vi "mecanum-drive-pose-est-test.vi"(8 "error in (no error)":errorcluster) -> (0 "error out":errorcluster, 3 "Test Passed":bool)   [LabVIEW 2019]
uses:
  <vilib>/Rock Robotics/WPI/ThirdParty/JAS_Junk/TrajLib/MatBuilder_Create.vi
  <vilib>/Rock Robotics/WPI/ThirdParty/JAS_Junk/TrajLib/MatrixHelper_CoerceSize.vi
  <vilib>/Rock Robotics/WPI/ThirdParty/JAS_Junk/TrajLib/Util_CalcDist.vi
  <vilib>/Analysis/1siggen.llb/Gaussian White Noise.vi
  <vilib>/Rock Robotics/WPI/ThirdParty/JAS_Junk/TrajLib/Trajectory_Library.lvlib
panel:
  out "BenchProcessing Timer Per Pass":dbl
  out "BenchTotalTime":dbl
  out "BenchTotalPasses":dbl
  out "MaxErrPassed":bool
  out "TotalPassed":bool
  out "EerrSumNormalized":dbl
  out "Error Sum":dbl
  out "Max Error":dbl
  out "Using Vision":bool
  in  "UseVIsion":bool=TRUE
  out "VIsionUpdates":i32
  out "TotalTImeSecs":dbl
  out "Position Graph":cluster{dbl[], dbl[]}[](graph)
  out "PoesEstCreateErr":errorcluster
  # "< 0.42"
  # "< 0.25"
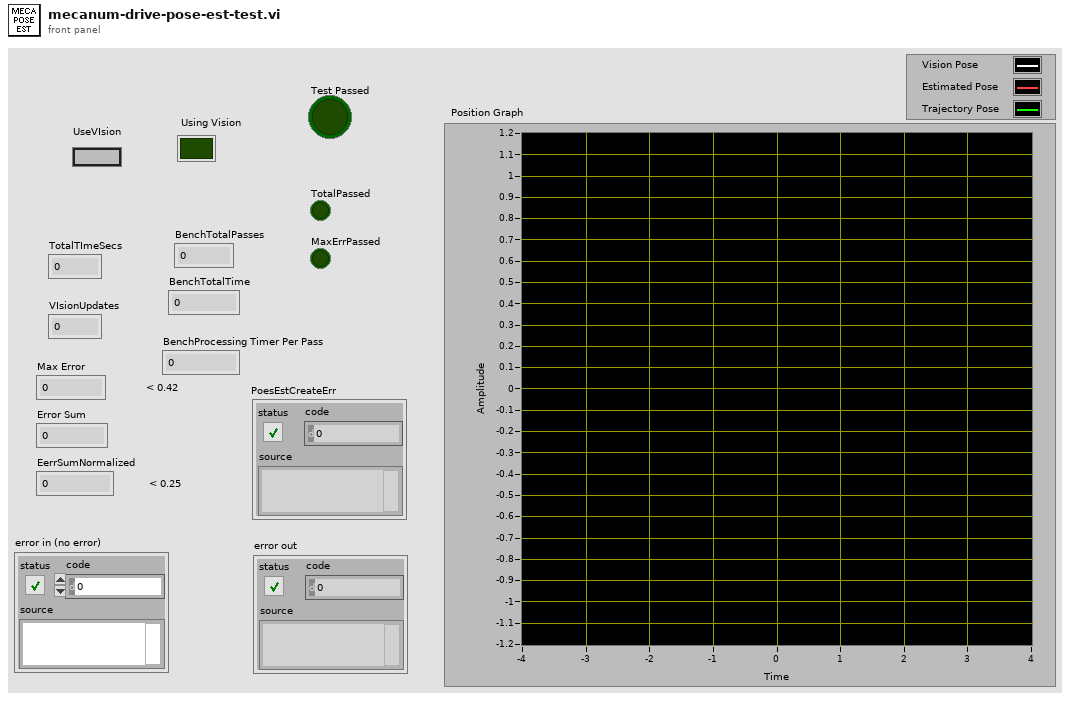
[diagram p1: front panel]
types:
  T1 = typedef "Trajectory_Library.lvlib/TRANSLATION2D.ctl" = cluster{"X":dbl, "Y":dbl}
  T2 = typedef "Trajectory_Library.lvlib/ROTATION2D.ctl" = cluster{"VALUE":dbl, "COS":dbl, "SIN":dbl}
  T3 = typedef "Trajectory_Library.lvlib/POSE2D.ctl" = cluster{"TRANSLATION":T1, "ROTATION":T2}
  T4 = typedef "NI_Matrix.lvlib/RealMatrix.ctl" = dbl[][]
  T5 = typedef "Trajectory_Library.lvlib/MECA_DRIVE_KINEMATICS.ctl" = cluster{"FrontLeft":T1, "FrontRight":T1, "RearLeft":T1, "RearRight":T1, "InverseKinematics":T4, "ForwardKinematics":T4, "PrevCoR":T1}
  T6 = typedef "Trajectory_Library.lvlib/TRAJ_CONFIG.ctl" = cluster{"MaxVelocity":dbl, "Max Acceleration":dbl, "StartVelocity":dbl, "End Velocity":dbl, "Reversed":bool, "DiffDrKineConstntDefined":bool, "CentAcellConstntDefined":bool, "DiffDrVoltConstntDefined":bool, "DIFF_DRIVE_KINE_CONSTRAINT":T7, "CENTRIPETAL_ACCEL_CONSTRAINT":T9, "SwerveDrKineConstntDefined":bool, "SWERVE_DRIVE_KINE_CONSTRAINT":T10, "DIFF_DRIVE_VOLTAGE_CONSTRAINT":T12, "MECANUM_DRIVE_KINE_CONSTRAINT":T14, "MecanumDrKineConstntDefined":bool}
  T7 = typedef "Trajectory_Library.lvlib/TRAJ_CONSTRAINT_DIIF_DRIVE_KINEMATICS.ctl" = cluster{"Max Speed (M/S)":dbl, "DIFF_DRIVE_KINEMATICS":T8, "Max Accel (M/S2)":dbl}
  T8 = typedef "Trajectory_Library.lvlib/DIFF_DRIVE_KINEMATICS.ctl" = cluster{"TrackWidth_Meters":dbl}
  T9 = typedef "Trajectory_Library.lvlib/TRAJ_CONSTRAINT_CENTRIPETAL_ACCEL.ctl" = cluster{"Max Cent Accel":dbl}
  T10 = typedef "Trajectory_Library.lvlib/TRAJ_CONSTRAINT_SWERVE_DRIVE_KINEMATICS.ctl" = cluster{"Max Speed (M/S)":dbl, "SwerveKinematics":T11}
  T11 = typedef "Trajectory_Library.lvlib/SWERVE_DRIVE_KINEMATICS.ctl" = cluster{"NumModules":i32, "InverseKinematics":T4, "ForwardKinematics":T4, "Modules":T1[], "PrevCoR":T1}
  T12 = typedef "Trajectory_Library.lvlib/TRAJ_CONSTRAINT_DIIF_DRIVE_VOLTAGE.ctl" = cluster{"Max Voltage":dbl, "DIFF_DRIVE_KINEMATICS":T8, "SIMPLE_MOTOR_FF":T13}
  T13 = typedef "Trajectory_Library.lvlib/SIMPLE_MOTOR_FF.ctl" = cluster{"Ks":dbl, "Kv":dbl, "Ka":dbl}
  T14 = typedef "Trajectory_Library.lvlib/TRAJ_CONSTRAINT_MECA_DRIVE_KINEMATICS.ctl" = cluster{"Max Speed (M/S)":dbl, "MECA_DRIVE_KINEMATICS":T5}
  T15 = typedef "Trajectory_Library.lvlib/MECA_DRIVE_POSE_EST.ctl" = cluster{"M_VisionContR":T4, "m_nominal_dT":dbl, "m_PrevTime_Sec":dbl, "m_GyroOffset":T2, "m_PrevAngle":T2, "m_Observer":T16, "m_kinematics":T5, "Pose_Buffer":T19}
  T16 = typedef "Trajectory_Library.lvlib/UNSCENTED_KALMAN_FILTER.ctl" = cluster{"m_P":T4, "m_xHat":T4, "States":i32, "Outputs":i32, "m_ContR":T4, "m_ContQ":T4, "m_SigmasF":T4, "m_dT_Sec":dbl, "MERWE_SCALED_SIGMA_PTS":T17, "meanFuncX":T18, "meanFuncY":T18, "residualFuncX":T18, "residualFuncY":T18, "addFuncX":T18, "addFuncXExtra":variant, "residualFuncYExtra":variant, "residualFuncXExtra":variant, "MeanFuncYExtra":variant, "MeanFuncXExtra":variant, "Inputs":i32}
  T17 = typedef "Trajectory_Library.lvlib/MERWE_SCALED_SIGMA_PTS.ctl" = cluster{"m_Wm":T4, "States":i32, "Alpha":dbl, "m_Wc":T4, "Kappa":i32}
  T18 = typedef "Trajectory_Library.lvlib/CALLBACK_FUNC_TYPE.ctl" = refnum<vi>
  T19 = typedef "Trajectory_Library.lvlib/TIME_INTERPOLATABLE_POSE.ctl" = cluster{"TimeStamps":dbl[], "Pose":T3[], "Min_TimeStamp":dbl, "Max_TimeStamp":dbl, "ItemCount":i32, "MaxBufferTime":dbl}
  T20 = typedef "Trajectory_Library.lvlib/TRAJECTORY.ctl" = cluster{"TotalTImeSecs":dbl, "States":T21[]}
  T21 = typedef "Trajectory_Library.lvlib/TRAJ_STATE.ctl" = cluster{"TimeSeconds":dbl, "Velocity":dbl, "Acceleration":dbl, "POSE":T3, "Curvature":dbl}
  T22 = typedef "Trajectory_Library.lvlib/CHASSIS_SPEEDS.ctl" = cluster{"vX":dbl, "vY":dbl, "vOmega":dbl}
  T23 = typedef "Trajectory_Library.lvlib/MECA_WHEEL_SPEEDS.ctl" = cluster{"FrontLeftSpeed":dbl, "FrontRightSpeed":dbl, "RearLeftSpeed":dbl, "RearRightSpeed":dbl}
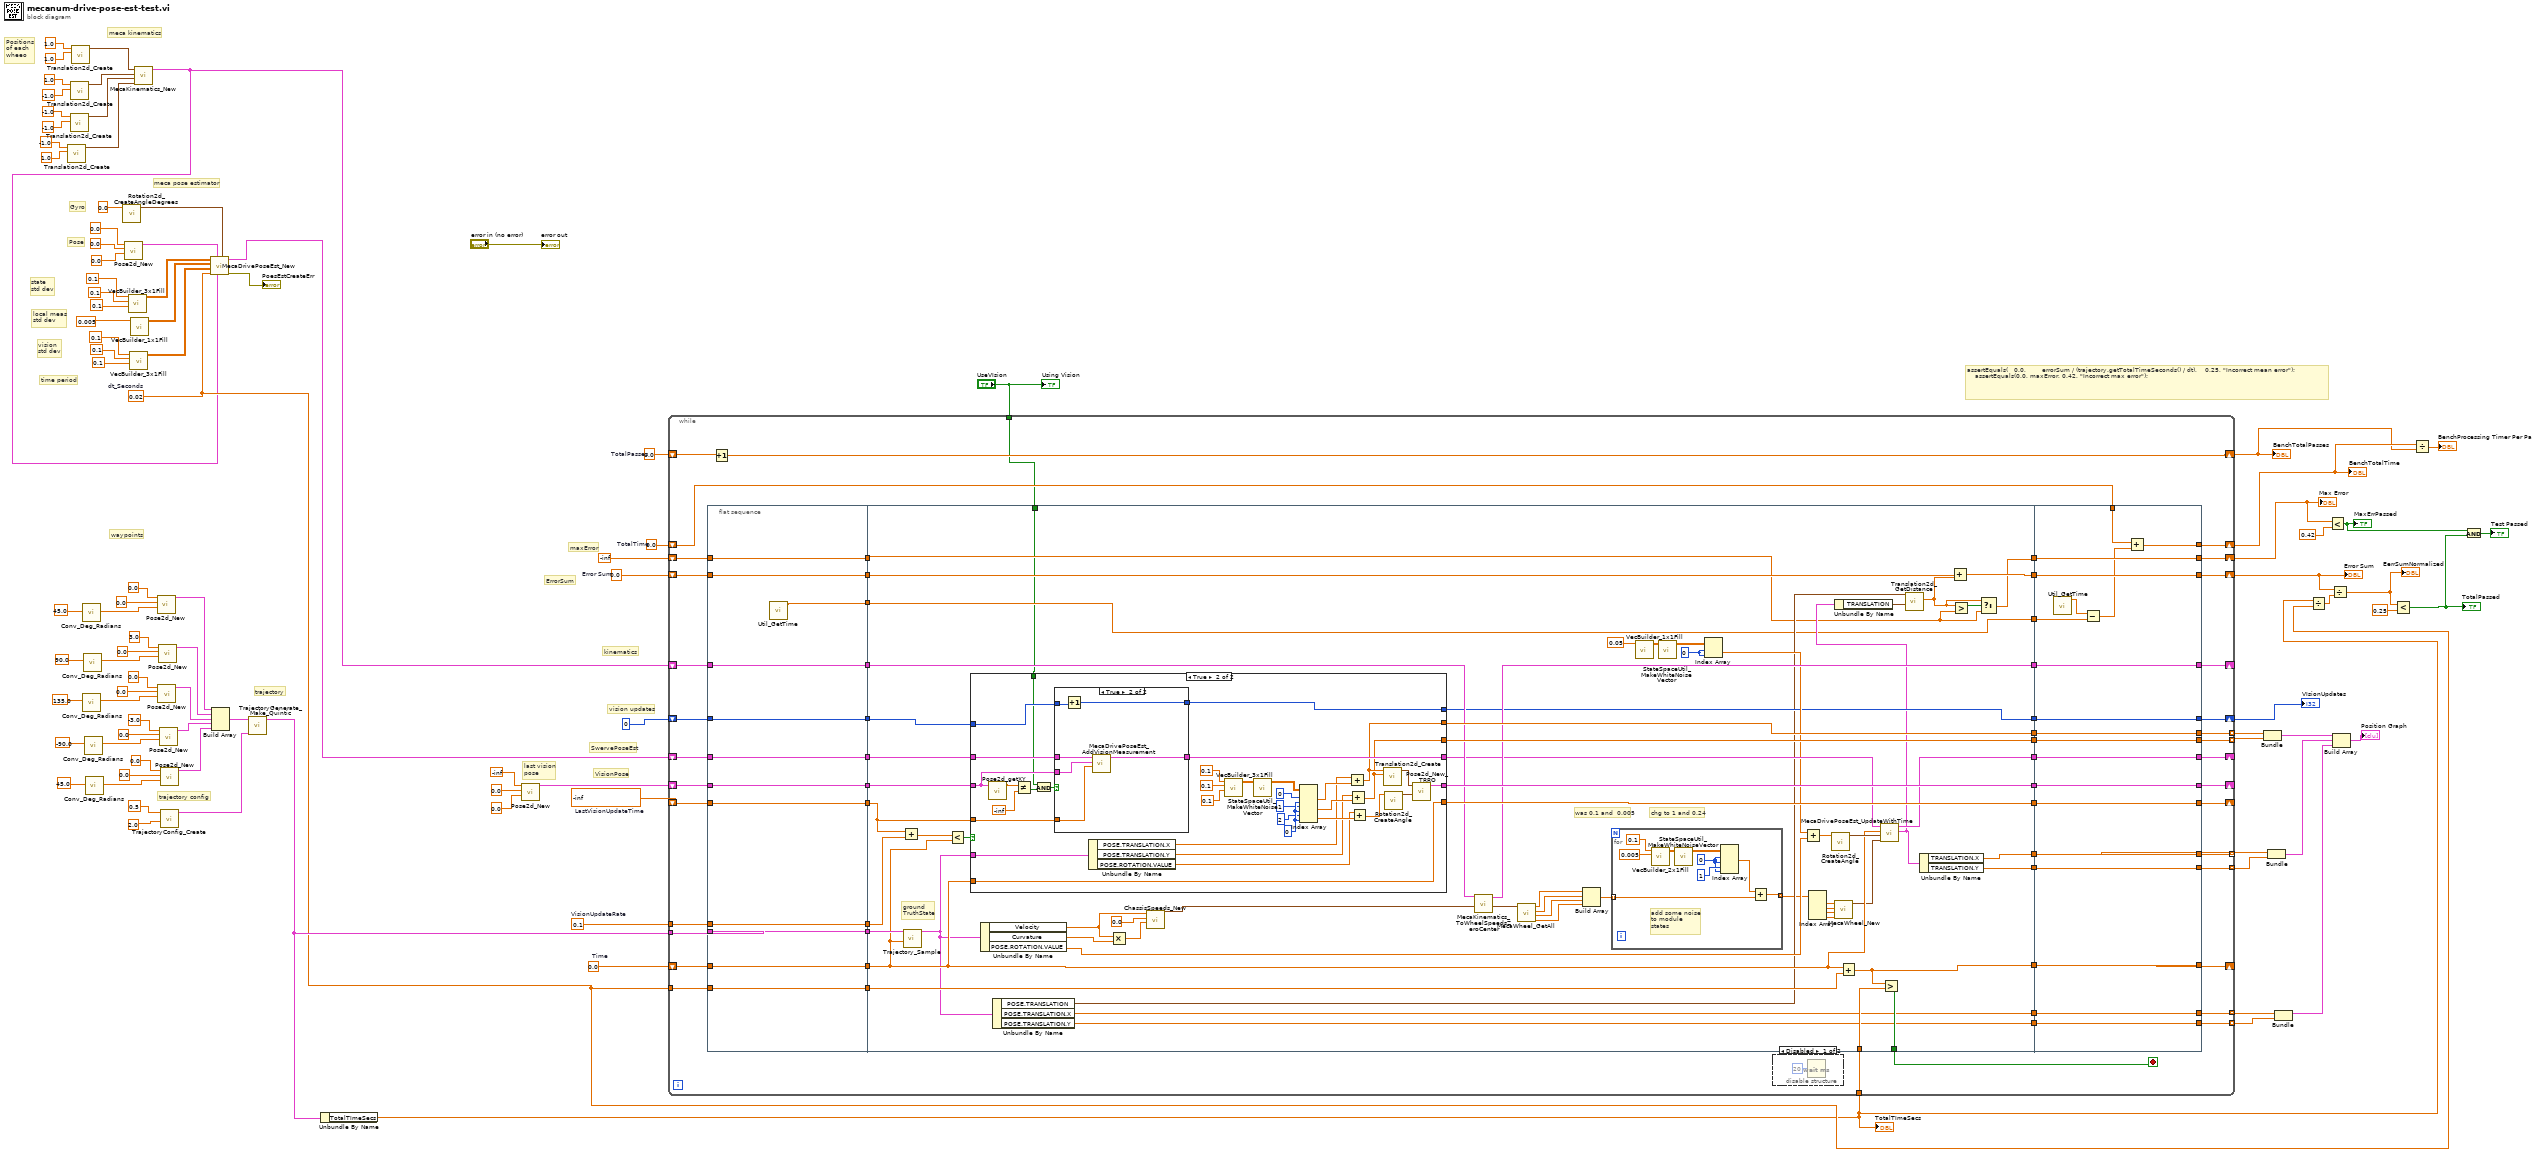
[diagram p0: block diagram]
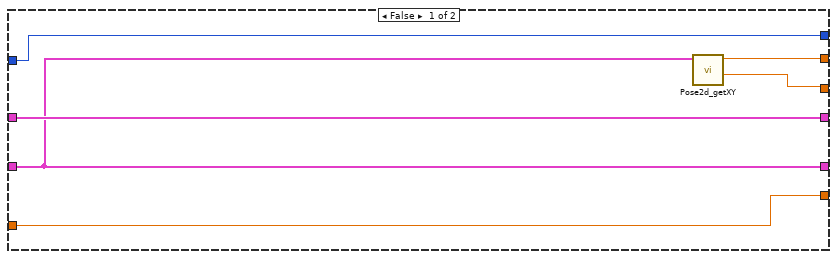
[diagram p3: hidden frame]
diagram:
  w8 = 0.0  # TotalPasses
  w9 = 0.0  # TotalTime
  w21 = 0.0  # Error Sum
  w39 = 0.1  # VisionUpdateRate
  w40 = -inf  # LastVisionUpdateTime
  w42 = 0.0  # Time
  w19 = 0.02  # dt_Seconds
  # "assertEquals(   0.0,        errorSum / (trajectory.getTotalTimeSeconds() / dt),    0.25, \"Incorrect mean error\");\n    assertEquals(0.0, maxError, 0.42, \"Incorrect max error\");"
  # "ErrorSum"
  # "maxError"
  # "vision updates"
  # "kinematics"
  # "SwervePoseEst"
  # "VisionPose"
  # "last vision\npose"
  # "time period"
  # "vision \nstd dev"
  # "local meas\nstd dev"
  # "state\nstd dev"
  # "Pose"
  # "Gyro"
  # "Positions\nof each\nwheeo"
  # "meca pose estimator"
  # "meca kinematics"
  # "trajectory config"
  # "trajectory"
  # "waypoints"
  n1 = call <vilib>:"Translation2d_Create.vi"("Y"=1.0, "X"=-1.0) -> ("TRANSLATION"=w60:T1)  [unwired: 9 in]
  n2 = call <vilib>:"Translation2d_Create.vi"("Y"=-1.0, "X"=-1.0) -> ("TRANSLATION"=w61:T1)  [unwired: 9 in]
  n3 = call <vilib>:"Translation2d_Create.vi"("Y"=-1.0, "X"=1.0) -> ("TRANSLATION"=w62:T1)  [unwired: 9 in]
  n4 = call <vilib>:"Translation2d_Create.vi"("Y"=1.0, "X"=1.0) -> ("TRANSLATION"=w63:T1)  [unwired: 9 in]
  n5 = call <vilib>:"Conv_Deg_Radians.vi"("Degress"=45.0 ("Heading")) -> ("Radians"=w77:dbl)  [unwired: 10 in]
  n6 = call <vilib>:"Conv_Deg_Radians.vi"("Degress"=135.0 ("Heading")) -> ("Radians"=w85:dbl)  [unwired: 10 in]
  n7 = call <vilib>:"Conv_Deg_Radians.vi"("Degress"=90.0 ("Heading")) -> ("Radians"=w81:dbl)  [unwired: 10 in]
  n8 = call <vilib>:"Conv_Deg_Radians.vi"("Degress"=-90.0 ("Heading")) -> ("Radians"=w89:dbl)  [unwired: 10 in]
  n9 = call <vilib>:"Conv_Deg_Radians.vi"("Degress"=45.0 ("Heading")) -> ("Radians"=w93:dbl)  [unwired: 10 in]
  n10 = call <vilib>:"Rotation2d_CreateAngleDegrees.vi"("Angle_Degrees"=0.0) -> ("ROTATION"=w59:T2)  [unwired: 10 in]
  n11 = call <vilib>:"Pose2d_New.vi"("Heading"=0.0, "Y"=0.0, "X"=0.0) -> ("out POSe"=w57:T3)  [unwired: 8 in]
  n12 = call <vilib>:"VecBuilder_3x1Fill.vi"("R2"=0.1 ("element"), "R1"=0.1 ("element"), "R0"=0.1 ("element")) -> ("output matrix"=w49:T4)  [unwired: 8 in]
  n13 = call <vilib>:"VecBuilder_3x1Fill.vi"("R2"=0.1 ("element"), "R1"=0.1 ("element"), "R0"=0.1 ("element")) -> ("output matrix"=w44:T4)  [unwired: 8 in]
  n14 = call <vilib>:"VecBuilder_1x1Fill.vi"("R0_C0"=0.005 ("element")) -> ("output matrix"=w48:T4)  [unwired: 10 in]
  n15 = call <vilib>:"MecaKinematics_New.vi"("RearRight"=w60, "RearLeft"=w61, "FrontRight"=w62, "FrontLeft"=w63) -> ("MECA_DRIVE_KINEMATICS"=w1:T5)  [unwired: 7 in]
  n16 = call <vilib>:"Pose2d_New.vi"("Heading"=w77, "Y"=0.0, "X"=0.0) -> ("out POSe"=w76:T3)  [unwired: 8 in]
  n17 = call <vilib>:"Pose2d_New.vi"("Heading"=w85, "Y"=0.0, "X"=0.0) -> ("out POSe"=w73:T3)  [unwired: 8 in]
  n18 = call <vilib>:"Pose2d_New.vi"("Heading"=w81, "Y"=0.0, "X"=3.0) -> ("out POSe"=w74:T3)  [unwired: 8 in]
  n19 = call <vilib>:"Pose2d_New.vi"("Heading"=w89, "Y"=0.0, "X"=-3.0) -> ("out POSe"=w72:T3)  [unwired: 8 in]
  n20 = call <vilib>:"Pose2d_New.vi"("Heading"=w93, "Y"=0.0, "X"=0.0) -> ("out POSe"=w98:T3)  [unwired: 8 in]
  n21 = call <vilib>:"TrajectoryConfig_Create.vi"("MaxAcceleration"=2.0, "MaxVelocity"=0.5) -> ("TRAJECTORY_CONFIG"=w95:T6)  [unwired: 9 in]
  n22 = call <vilib>:"MecaDrivePoseEst_New.vi"("gyroAngle"=w59, "MecanumKinematics"=w1, "InitialPose"=w57, "dt_Seconds"=w19, "VisionMeasurementStdDevs"=w44, "LocalMeasurementStdDevs"=w48, "StateStdDevs"=w49) -> ("Error"=→"PoesEstCreateErr":errorcluster, "MecaDrivePoseEstimate"=w2:T15)  [unwired: 3 in]
  n23 = Build Array(w76, w74, w73, w72, w98) -> (w96:T3[])
  n24 = call <vilib>:"TrajectoryGenerate_Make_Quintic.vi"("traj_config"=w95, "waypointPOSE"=w96) -> ("TRAJECTORY"=w41:T20)  [unwired: 8 in, 1 out]
  n25 = Unbundle By Name(w41) -> ("TotalTImeSecs"=w12:dbl)
  "TotalTImeSecs" <- w12
  n26 = call <vilib>:"Pose2d_New.vi"("Heading"=0.0, "Y"=0.0, "X"=-inf) -> ("out POSe"=w35:T3)  [unwired: 8 in]
  n27 = while {
    tunnel: w19 -> [w159]
    shift-right: [w158] -> _
    shift-left: w42 -> [w145]
    tunnel: w41 -> [w156]
    tunnel: w12 -> [w157]
    shift-right: [w150] -> _
    shift-left: w40 -> [w152]
    tunnel: w39 -> [w155]
    shift-right: [w151] -> _
    shift-left: w35 -> [w154]
    shift-right: [w144] -> _
    shift-left: w2 -> [w153]
    tunnel: [w149] -> w34 mode=indexing
    tunnel: [w148] -> w33 mode=indexing
    shift-right: [w146] -> _
    shift-left: w1 -> [w147]
    tunnel: [w143] -> w32 mode=indexing
    tunnel: [w142] -> w31 mode=indexing
    shift-right: [w140] -> w26
    shift-left: 0 -> [w141]
    tunnel: [w139] -> w25 mode=indexing
    tunnel: [w138] -> w24 mode=indexing
    shift-right: [w135] -> w17
    shift-left: -inf -> [w134]
    shift-right: [w136] -> w20
    shift-left: w21 -> [w137]
    shift-right: [w105] -> w7
    shift-left: w9 -> [w104]
    shift-right: [w102] -> w6
    shift-left: w8 -> [w103]
    tunnel: "UseVIsion" -> [w101]
    stop <- w133 stop-if-true
    n28 = flat-sequence {
      tunnel: w134 -> [w162]
      tunnel: w137 -> [w163]
      tunnel: w141 -> [w164]
      tunnel: w145 -> [w165]
      tunnel: w147 -> [w166]
      tunnel: w152 -> [w167]
      tunnel: w153 -> [w168]
      tunnel: w154 -> [w169]
      tunnel: w155 -> [w170]
      tunnel: w156 -> [w171]
      tunnel: w159 -> [w172]
      tunnel: [w172] -> w132
      tunnel: [w171] -> w131
      tunnel: [w170] -> w130
      tunnel: [w169] -> w129
      tunnel: [w168] -> w128
      tunnel: [w167] -> w127
      tunnel: [w166] -> w126
      tunnel: [w165] -> w125
      tunnel: [w164] -> w124
      tunnel: [w163] -> w123
      tunnel: [w162] -> w122
      tunnel: [w161] -> w107
      tunnel: [w234] -> w133
      tunnel: w157 -> [w232]
      tunnel: w132 -> [w235]
      tunnel: w131 -> [w231]
      tunnel: w130 -> [w229]
      tunnel: w129 -> [w227]
      tunnel: w128 -> [w226]
      tunnel: w127 -> [w225]
      tunnel: w126 -> [w215]
      tunnel: w125 -> [w204]
      tunnel: w124 -> [w200]
      tunnel: w123 -> [w192]
      tunnel: w122 -> [w187]
      tunnel: [w233] -> w121
      tunnel: [w224] -> w120
      tunnel: [w223] -> w119
      tunnel: [w222] -> w118
      tunnel: [w221] -> w117
      tunnel: [w214] -> w116
      tunnel: [w203] -> w115
      tunnel: [w202] -> w114
      tunnel: [w201] -> w113
      tunnel: [w199] -> w112
      tunnel: [w197] -> w111
      tunnel: [w196] -> w110
      tunnel: [w191] -> w109
      tunnel: [w188] -> w108
      tunnel: w107 -> [w186]
      tunnel: [w186] -> w106
      tunnel: w101 -> [w185]
      tunnel: [w298] -> w135
      tunnel: [w299] -> w136
      tunnel: [w300] -> w138
      tunnel: [w301] -> w139
      tunnel: [w302] -> w140
      tunnel: [w303] -> w142
      tunnel: [w304] -> w143
      tunnel: [w305] -> w144
      tunnel: [w306] -> w146
      tunnel: [w307] -> w148
      tunnel: [w308] -> w149
      tunnel: [w309] -> w150
      tunnel: [w310] -> w151
      tunnel: [w311] -> w158
      tunnel: w121 -> [w311]
      tunnel: w120 -> [w310]
      tunnel: w119 -> [w309]
      tunnel: w118 -> [w308]
      tunnel: w117 -> [w307]
      tunnel: w116 -> [w306]
      tunnel: w115 -> [w305]
      tunnel: w114 -> [w304]
      tunnel: w113 -> [w303]
      tunnel: w112 -> [w302]
      tunnel: w111 -> [w301]
      tunnel: w110 -> [w300]
      tunnel: w109 -> [w299]
      tunnel: w108 -> [w298]
      tunnel: w106 -> [w296]
      tunnel: [w295] -> w105
      tunnel: w104 -> [w293]
      frame #0 {
        n29 = call <vilib>:"Util_GetTime.vi"() -> ("FPGA_Time_Seconds"=w161:dbl)  [unwired: 10 in, 1 out]
      }
      frame #1 {
        w209 = 0 ("index (col)")
        # "chg to 1 and 0.24"
        # "was 0.1 and  0.005"
        # "ground\nTruthState"
        n30 = Add(x=w225, y=w229) -> (x+y=w228:dbl)
        n31 = call <vilib>:"Trajectory_Sample.vi"("Time"=w204, "InputTRAJECTORY"=w231) -> ("OutputTRAJ_STATE"=w198:T21)  [unwired: 9 in]
        n32 = Less?(x=w228, y=w204) -> (x < y?=w230:bool)
        n33 = case shown="True" w230 {
          tunnel: w227 -> [w248 w281]
          tunnel: w226 -> [w250 w282]
          tunnel: [w250 w280] -> w213
          tunnel: w225 -> [w249 w279]
          tunnel: w198 -> [_ w272]
          tunnel: [w248 w278] -> w224
          tunnel: w204 -> [_ w258]
          tunnel: [w249 w258] -> w223
          tunnel: [w247 w257] -> w222
          tunnel: [w246 w256] -> w221
          tunnel: w200 -> [w245 w255]
          tunnel: [w245 w254] -> w199
          tunnel: w185 -> [_ w251]
          frame False {
            n34 = call <vilib>:"Pose2d_getXY.vi"("in POSE"=w248) -> ("Y"=w246:dbl, "X"=w247:dbl)  [unwired: 9 in]
          }
          frame True {
            w269 = 0 ("index (col)")
            n35 = call <vilib>:"Pose2d_getXY.vi"("in POSE"=w281) -> ("X"=w284:dbl)  [unwired: 9 in, 1 out]
            n36 = Not Equal?(x=w284, y=-inf) -> (x != y?=w252:bool)
            n37 = And(x=w251, y=w252) -> (x .and. y?=w253:bool)
            n38 = case shown="True" w253 {
              tunnel: w282 -> [w286 w292]
              tunnel: w281 -> [_ w291]
              tunnel: [w286 w290] -> w280
              tunnel: w279 -> [_ w289]
              tunnel: w255 -> [w285 w288]
              tunnel: [w285 w287] -> w254
              frame False {
              }
              frame True {
                n39 = Increment(x=w288) -> (x+1=w287:i32)
                n40 = call <vilib>:"MecaDrivePoseEst_AddVisionMeasurement.vi"("TImeStamp_Seconds"=w289, "visionRobotPose"=w291, "in MecaDrivePoseEstimate"=w292) -> ("OutMecaDrivePoseEstimate"=w290:T15)  [unwired: 7 in, 1 out]
              }
            }
            n41 = Unbundle By Name(w272) -> ("POSE.TRANSLATION.X"=w261:dbl, "POSE.TRANSLATION.Y"=w260:dbl, "POSE.ROTATION.VALUE"=w259:dbl)
            n42 = call <vilib>:"VecBuilder_3x1Fill.vi"("R2"=0.1, "R1"=0.1, "R0"=0.1) -> ("output matrix"=w276:T4)  [unwired: 8 in]
            n43 = call <vilib>:"StateSpaceUtil_MakeWhiteNoiseVector.vi"("StdDevs"=w276) -> ("WhiteNoise"=w270:T4)  [unwired: 9 in, 1 out]
            n44 = Index Array(array=w270, index (row) #1=0 ("index (col)"), index (col) #1=w269, index (row) #2=1 ("index (col)"), index (col) #2=w269, index (row) #3=2 ("index (col)"), index (col) #3=w269) -> (element #1=w263:dbl, element #2=w264:dbl, element #3=w265:dbl)
            n45 = Add(x=w261, y=w263) -> (x+y=w257:dbl)
            n46 = Add(x=w260, y=w264) -> (x+y=w256:dbl)
            n47 = Add(x=w259, y=w265) -> (x+y=w262:dbl)
            n48 = call <vilib>:"Translation2d_Create.vi"("Y"=w256, "X"=w257) -> ("TRANSLATION"=w277:T1)  [unwired: 9 in]
            n49 = call <vilib>:"Rotation2d_CreateAngle.vi"("Angle"=w262) -> ("ROTATION"=w271:T2)  [unwired: 10 in]
            n50 = call <vilib>:"Pose2d_New_TRRO.vi"("ROTATION"=w271, "TRANSLATION"=w277) -> ("outPOSE"=w278:T3)  [unwired: 9 in]
          }
        }
        n51 = Unbundle By Name(w198) -> ("Velocity"=w218:dbl, "Curvature"=w219:dbl, "POSE.ROTATION.VALUE"=w208:dbl)
        n52 = Unbundle By Name(w198) -> ("POSE.TRANSLATION"=w195:T1, "POSE.TRANSLATION.X"=w196:dbl, "POSE.TRANSLATION.Y"=w197:dbl)
        n53 = Multiply(x=w218, y=w219) -> (x*y=w217:dbl)
        n54 = call <vilib>:"ChassisSpeeds_New.vi"("vAngular"=w217, "vY"=0.0, "vX"=w218) -> ("CHASSIS"=w216:T22)  [unwired: 8 in]
        n55 = call <vilib>:"MecaKinematics_ToWheelSpeedsZeroCenter.vi"("ChassisSpeeds"=w216, "in MECA_DRIVE_KINEMATICS"=w215) -> ("MECA_WHEEL_SPEEDS"=w184:T23, "out MECA_DRIVE_KINEMATICS"=w214:T5)  [unwired: 8 in]
        n56 = call <vilib>:"MecaWheel_GetAll.vi"("MECA_WHEEL_SPEEDS"=w184) -> ("RearRightSpeed"=w180:dbl, "RearLeftSpeed"=w181:dbl, "FrontRightSpeed"=w182:dbl, "FrontLeftSpeed"=w183:dbl)  [unwired: 7 in]
        n57 = Build Array(w183, w182, w181, w180) -> (w179:dbl[])
        n58 = for {
          tunnel: [w236] -> w178 mode=indexing
          tunnel: w179 -> [w237] mode=indexing
          w239 = 0 ("index (col)")
          # "add some noise\nto module\nstates"
          n59 = call <vilib>:"VecBuilder_2x1Fill.vi"("R1"=0.005, "R0"=0.1) -> ("output matrix"=w244:T4)  [unwired: 9 in]
          n60 = call <vilib>:"StateSpaceUtil_MakeWhiteNoiseVector.vi"("StdDevs"=w244) -> ("WhiteNoise"=w241:T4)  [unwired: 9 in, 1 out]
          n61 = Index Array(array=w241, index (row) #1=w239, index (col) #1=w239, index (row) #2=1 ("index (col)"), index (col) #2=w239) -> (element #1=w238:dbl)  [unwired: 1 out]
          n62 = Add(x=w238, y=w237) -> (x+y=w236:dbl)
        }
        n63 = call <vilib>:"VecBuilder_1x1Fill.vi"("R0_C0"=0.05 ("R0")) -> ("output matrix"=w212:T4)  [unwired: 10 in]
        n64 = call <vilib>:"StateSpaceUtil_MakeWhiteNoiseVector.vi"("StdDevs"=w212) -> ("WhiteNoise"=w210:T4)  [unwired: 9 in, 1 out]
        n65 = Index Array(array=w210, index (row)=w209, index (col)=w209) -> (element=w207:dbl)
        n66 = Add(x=w207, y=w208) -> (x+y=w206:dbl)
        n67 = Index Array(array=w178) -> (element #1=w176:dbl, element #2=w175:dbl, element #3=w174:dbl, element #4=w173:dbl)  [unwired: 4 in]
        n68 = call <vilib>:"Rotation2d_CreateAngle.vi"("Angle"=w206) -> ("ROTATION"=w205:T2)  [unwired: 10 in]
        n69 = call <vilib>:"MecaWheel_New.vi"("RearRightSpeed"=w173, "RearLeftSpeed"=w174, "FrontRightSpeed"=w175, "FrontLeftSpeed"=w176) -> ("MECA_WHEEL_SPEEDS"=w177:T23)  [unwired: 7 in]
        n70 = Add(x=w204, y=w235) -> (x+y=w233:dbl)
        n71 = call <vilib>:"MecaDrivePoseEst_UpdateWithTime.vi"("MecanumWheelSpeeds"=w177, "GyroAngle"=w205, "CurrentTimeSeconds"=w204, "in MecaDrivePoseEstimate"=w213) -> ("Estimated Pose"=w194:T3, "Out MecaDrivePoseEstimate"=w203:T15)  [unwired: 5 in, 1 out]
        n72 = Unbundle By Name(w194) -> ("TRANSLATION"=w193:T1)
        n73 = Greater?(x=w233, y=w232) -> (0:w234:bool)
        n74 = call <vilib>:"Translation2d_GetDistance.vi"("other Translation"=w193, "In Translation"=w195) -> ("Distance"=w189:dbl)  [unwired: 9 in]
        n75 = Unbundle By Name(w194) -> ("TRANSLATION.X"=w202:dbl, "TRANSLATION.Y"=w201:dbl)
        n76 = Add(x=w192, y=w189) -> (x+y=w191:dbl)
        n77 = Greater?(x=w189, y=w187) -> (0:w190:bool)
        n78 = Select(t=w189, s=w190, f=w187) -> (s? t:f=w188:dbl)
      }
      frame #2 {
        n79 = call <vilib>:"Util_GetTime.vi"() -> ("FPGA_Time_Seconds"=w297:dbl)  [unwired: 10 in, 1 out]
        n80 = Subtract(x=w297, y=w296) -> (x-y=w294:dbl)
        n81 = Add(x=w293, y=w294) -> (x+y=w295:dbl)
      }
    }
    n82 = Increment(x=w103) -> (x+1=w102:dbl)
    n83 = disable-structure shown="Disabled" {
      frame Disabled {
        n84 = Wait (ms)(milliseconds to wait=u32 20) -> ()  [unwired: 1 out]
      }
      frame Enabled {
      }
    }
  }
  "VIsionUpdates" <- w26
  "Max Error" <- w17
  "Error Sum" <- w20
  "BenchTotalPasses" <- w6
  "BenchTotalTime" <- w7
  n85 = Bundle(w34, w33) -> (w30:cluster{dbl[], dbl[]})  [unwired: 1 in]
  n86 = Bundle(w32, w31) -> (w29:cluster{dbl[], dbl[]})  [unwired: 1 in]
  n87 = Bundle(w24, w25) -> (w23:cluster{dbl[], dbl[]})  [unwired: 1 in]
  n88 = Divide(x=w12, y=w19) -> (x/y=w10:dbl)
  n89 = Less?(x=w17, y=0.42) -> (x < y?=w15:bool)
  "MaxErrPassed" <- w15
  n90 = Divide(x=w20, y=w10) -> (x/y=w11:dbl)
  "EerrSumNormalized" <- w11
  n91 = Build Array(w30, w29, w23) -> (→"Position Graph":cluster{dbl[], dbl[]}[])
  n92 = Less?(x=w11, y=0.25) -> (x < y?=w14:bool)
  "TotalPassed" <- w14
  n93 = Divide(x=w7, y=w6) -> (x/y=→"BenchProcessing Timer Per Pass":dbl)
  n94 = And(x=w15, y=w14) -> (x .and. y?=→"Test Passed":bool)
  "Using Vision" <- "UseVIsion"
  "error out" <- "error in (no error)"
